vi "Measurement UI.vi"() -> ()   [LabVIEW 2024, in "Tone Generation UI.lvlib"]
uses:
  Tone Generation UI.lvlib
  <vilib>/Utility/error.llb/Trim Whitespace One-Sided.vi
panel:
  in  "sample rate":dbl=51200.0 min=100.0 max=1000000.0 step=100.0 format="%#_g Hz"
  in  "physical channels":string[](array[string])
  in  "phases":dbl[](array[numeric])
  in  "amplitudes":dbl[](array[numeric])
  in  "frequencies":dbl[](array[numeric])
  in  "terminal cfgs":i32[](array[numeric])
  in  "ranges":dbl[](array[numeric])
  in  "output configurations":T1(array[cluster])=[{"channel"="Dev1/ao0", "range"=3.16, "terminal configuration"=-1, "frequency"=997.0, "amplitude"=1.0, "phase"=0.0}, {"channel"="Dev1/ao1", "range"=3.16, "terminal configuration"=-1, "frequency"=997.0, "amplitude"=1.0, "phase"=90.0}] {"phase" min=-360.0 max=360.0 step=10.0 format="%#_g deg"; "amplitude" min=0.0 max=10.0 format="%_4g V"; "frequency" min=0.001 step=10.0 format="%#_4g Hz"; "terminal configuration" items=["Default"=-1, "RSE"=10083, "Differential"=10106, "Pseudodifferential"=12529]; "range" min=0.1 max=10.0 step=1.0 format="± %#_4g V"}
  out "error code out":i32
  out "error description out":string="Empty"
  out "error out":bool
  out "Task":u16(ring)
  out "generator status":string="Idle"
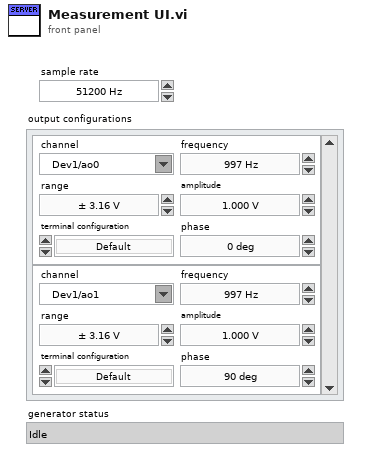
[diagram p1: front panel]
types:
  T1 = cluster{"channel":tag, "range":dbl, "terminal configuration":i32, "frequency":dbl, "amplitude":dbl, "phase":dbl}[]
  T2 = cluster{"channel":tag, "range":dbl, "terminal configuration":i32, "frequency":dbl, "amplitude":dbl, "phase":dbl}
  T3 = enum8{"Enabled", "Disabled", "Disabled and Grayed Out"}
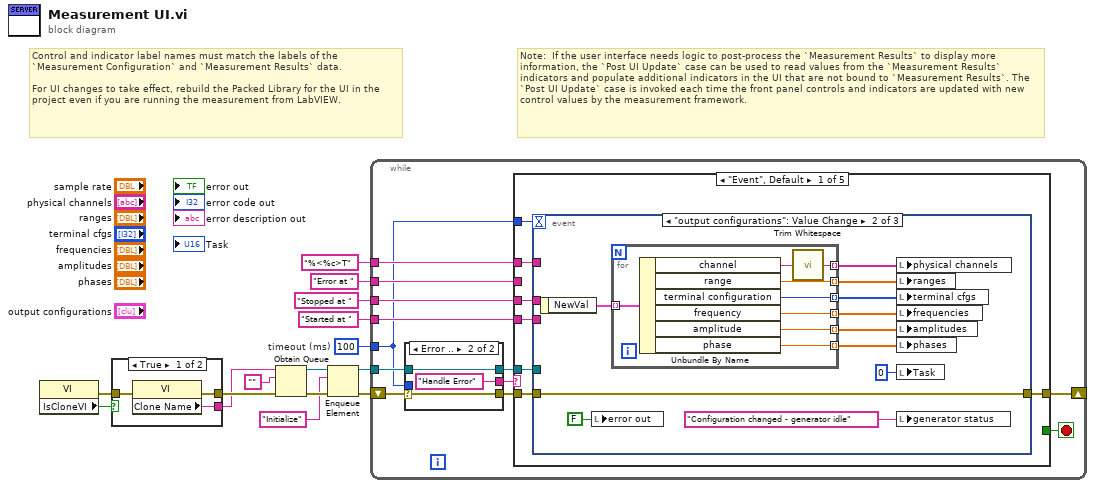
[diagram p0: block diagram]
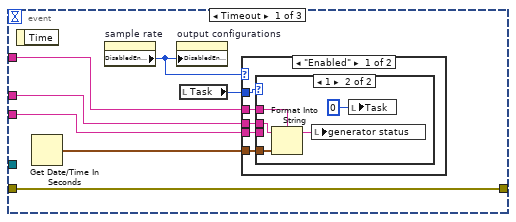
[diagram p2: hidden frame]
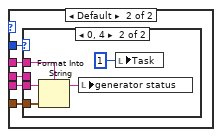
[diagram p4: hidden frame]
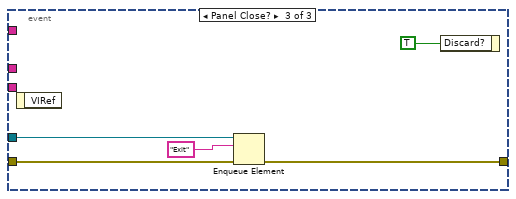
[diagram p6: hidden frame]
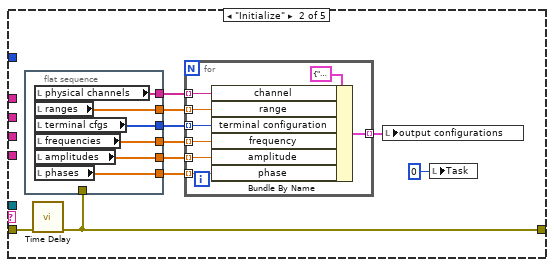
[diagram p7: hidden frame]
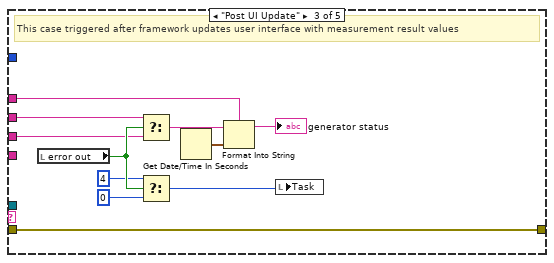
[diagram p8: hidden frame]
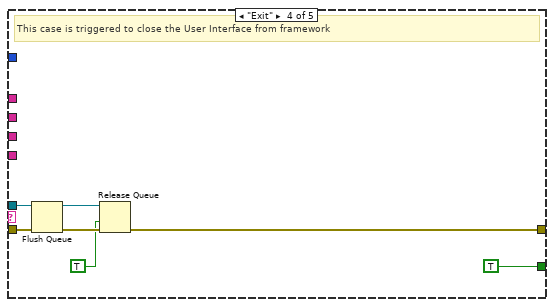
[diagram p9: hidden frame]
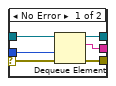
[diagram p11: hidden frame]
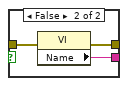
[diagram p12: hidden frame]
diagram:
  w1 = 100  # timeout (ms)
  # "Control and indicator label names must match the labels of the `Measurement Configuration` and `Measurement Results` data. \n\nFor UI changes to take effect, rebuild the Packed Library for the UI in the project even if you are running the measurement from LabVIEW."
  # "Note:  If the user interface needs logic to post-process the `Measurement Results` to display more information, the `Post UI Update` case can be used to read values from the `Measurement Results` indicators and populate additional indicators in the UI that are not bound to `Measurement Results`. The `Post UI Update` case is invoked each time the front panel controls and indicators are updated with new control values by the measurement framework."
  n1 = property class="VI"() -> (error out=w6:errorcluster, "IsCloneVI"=w7:bool)  [unwired: 2 in, 1 out]
  n2 = case shown="True" w7 {
    tunnel: [w18 w21] -> w15
    tunnel: [w17 w20] -> w14
    tunnel: w6 -> [w16 w19]
    frame True {
      n3 = property class="VI"(error in=w16) -> (error out=w18:errorcluster, "Clone Name"=w17:string)  [unwired: 1 in, 1 out]
    }
    frame False {
      n4 = property class="VI"(error in=w19) -> (error out=w21:errorcluster, "Name"=w20:string)  [unwired: 1 in, 1 out]
    }
  }
  n5 = Obtain Queue(name (unnamed)=w14, element data type="", error in (no error)=w15) -> (queue out=w11:refnum<queue>, error out=w13:errorcluster)  [unwired: 2 in, 1 out]
  n6 = Enqueue Element(queue=w11, element="Initialize", error in (no error)=w13) -> (queue out=w10:refnum<queue>, error out=w12:errorcluster)  [unwired: 1 in, 1 out]
  n7 = while {
    shift-right: [w28] -> _
    shift-left: w12 -> [w33]
    tunnel: w10 -> [w31]
    tunnel: "Started at " ("format string") -> [w26]
    tunnel: "Error at " ("current status") -> [w25]
    tunnel: "Stopped at " ("current status") -> [w24]
    tunnel: "%<%c>T" ("format string") -> [w23]
    tunnel: w1 -> [w22]
    stop <- w27 stop-if-true
    n8 = case shown="Error .." w33 {
      selector: w33 -> [w140 w143]
      tunnel: [w139 w143] -> w32
      tunnel: w31 -> [w138 w142]
      tunnel: [w137 w142] -> w30
      tunnel: [w136 "Handle Error"] -> w29
      tunnel: w22 -> [w135 _]
      frame No Error {
        n9 = Dequeue Element(queue=w138, timeout in ms (-1)=w135, error in (no error)=w140) -> (queue out=w137:refnum<queue>, element=w136:string, error out=w139:errorcluster)  [unwired: 1 out]
      }
      frame Error {
      }
    }
    n10 = case shown="\"Event\", Default" w29 {
      tunnel: w32 -> [w39 w100 w126 w133 w134]
      tunnel: w30 -> [w38 _ _ w131 _]
      tunnel: [w40 w92 w126 w128 w134] -> w28
      tunnel: [_ _ _ TRUE _] -> w27
      tunnel: w22 -> [w37 _ _ _ _]
      tunnel: w25 -> [_ _ w118 _ _]
      tunnel: w24 -> [w35 _ w117 _ _]
      tunnel: w26 -> [w36 _ _ _ _]
      tunnel: w23 -> [w34 _ w116 _ _]
      frame "Event", Default {
        n11 = event shown="[1] \"output configurations\": Value Change" {
          selector: _ -> [_ _ _]
          dyn-events: _ -> [_ _ _]
          timeout: w37 -> [_ _ _]
          tunnel: [w47 w78 w89] -> w40
          tunnel: w39 -> [w47 w78 w90]
          tunnel: w38 -> [_ _ w88]
          tunnel: w36 -> [w44 _ _]
          tunnel: w35 -> [w42 _ _]
          tunnel: w34 -> [w41 _ _]
          event Timeout {
            n12 = event-data() -> ()  [unwired: 1 in, 1 out]
            n13 = Get Date/Time In Seconds() -> (seconds since 1Jan1904=w43:timestamp)
            n14 = property on="sample rate" class="DigNum (strict)"() -> ("DisabledEnum"=w46:T3)  [unwired: 2 in, 2 out]
            n15 = property on="output configurations" class="Arr (strict)"("DisabledEnum"=w46) -> ()  [unwired: 2 in, 2 out]
            n16 = local read "Task"() -> (w45:u16)
            n17 = case shown="\"Enabled\"" w46 {
              tunnel: w45 -> [w52 w62]
              tunnel: w44 -> [w49 w61]
              tunnel: w41 -> [w51 w59]
              tunnel: w43 -> [w50 w60]
              tunnel: w42 -> [w48 w58]
              frame "Enabled" {
                n18 = case shown="1" w52 {
                  tunnel: w51 -> [_ w55]
                  tunnel: w50 -> [_ w54]
                  tunnel: w49 -> [_ _]
                  tunnel: w48 -> [_ w53]
                  frame Default {
                  }
                  frame 1 {
                    n19 = Format Into String(format string=w55, initial string=w53, w54) -> (resulting string=w57:string)  [unwired: 1 in, 1 out]
                    n20 = local write "generator status"(w57) -> ()
                    n21 = local write "Task"(u16 0 ("Task")) -> ()
                  }
                }
              }
              frame Default {
                n22 = case shown="0, 4" w62 {
                  tunnel: w61 -> [_ w65]
                  tunnel: w60 -> [_ w64]
                  tunnel: w59 -> [_ w63]
                  tunnel: w58 -> [_ _]
                  frame Default {
                  }
                  frame 0, 4 {
                    n23 = Format Into String(format string=w63, initial string=w65, w64) -> (resulting string=w67:string)  [unwired: 1 in, 1 out]
                    n24 = local write "generator status"(w67) -> ()
                    n25 = local write "Task"(u16 1 ("Task")) -> ()
                  }
                }
              }
            }
          }
          event "output configurations": Value Change {
            n26 = event-data() -> ("NewVal"=w71:T1)  [unwired: 1 in]
            n27 = local write "error out"(FALSE ("error out")) -> ()
            n28 = for {
              tunnel: w71 -> [w86] mode=indexing
              tunnel: [w79] -> w77 mode=indexing
              tunnel: [w85] -> w76 mode=indexing
              tunnel: [w84] -> w75 mode=indexing
              tunnel: [w83] -> w74 mode=indexing
              tunnel: [w82] -> w73 mode=indexing
              tunnel: [w81] -> w72 mode=indexing
              n29 = Unbundle By Name(w86) -> ("channel"=w80:tag, "range"=w85:dbl, "terminal configuration"=w84:i32, "frequency"=w83:dbl, "amplitude"=w82:dbl, "phase"=w81:dbl)
              n30 = call <vilib>:"Trim Whitespace.vi"("string"=w80) -> ("trimmed string"=w79:string)  [unwired: 1 in]
            }
            n31 = local write "physical channels"(w77) -> ()
            n32 = local write "ranges"(w76) -> ()
            n33 = local write "terminal cfgs"(w75) -> ()
            n34 = local write "frequencies"(w74) -> ()
            n35 = local write "amplitudes"(w73) -> ()
            n36 = local write "phases"(w72) -> ()
            n37 = local write "Task"(u16 0 ("Task")) -> ()
            n38 = local write "generator status"("Configuration changed - generator idle" ("current status")) -> ()
          }
          event Panel Close? {
            n39 = event-data() -> ()  [unwired: 1 in, 1 out]
            n40 = Enqueue Element(queue=w88, element="Exit", error in (no error)=w90) -> (error out=w89:errorcluster)  [unwired: 1 in, 2 out]
            n41 = event-data("Discard?"=TRUE) -> ()  [unwired: 1 in, 1 out]
          }
        }
      }
      frame "Initialize" {
        n42 = flat-sequence {
          tunnel: [w107] -> w99
          tunnel: [w106] -> w98
          tunnel: [w105] -> w97
          tunnel: [w104] -> w96
          tunnel: [w103] -> w95
          tunnel: [w102] -> w94
          tunnel: w92 -> [_]
          frame #0 {
            n43 = local read "physical channels"() -> (w107:string[])
            n44 = local read "ranges"() -> (w106:dbl[])
            n45 = local read "terminal cfgs"() -> (w105:i32[])
            n46 = local read "frequencies"() -> (w104:dbl[])
            n47 = local read "amplitudes"() -> (w103:dbl[])
            n48 = local read "phases"() -> (w102:dbl[])
          }
        }
        n49 = call "Time Delay"("error in (no error)"=w100) -> ("error out"=w92:errorcluster)  [unwired: 10 in]
        n50 = for {
          tunnel: w99 -> [w115] mode=indexing
          tunnel: w98 -> [w114] mode=indexing
          tunnel: w97 -> [w113] mode=indexing
          tunnel: w96 -> [w112] mode=indexing
          tunnel: w95 -> [w111] mode=indexing
          tunnel: w94 -> [w110] mode=indexing
          tunnel: [w108] -> w93 mode=indexing
          n51 = Bundle By Name(cluster=T2 {"channel"="Dev1/ao0", "range"=3.16, "terminal configuration"=-1, "frequency"=997.0, "amplitude"=1.0, "phase"=0.0} ("output configuration"), "channel"=w115, "range"=w114, "terminal configuration"=w113, "frequency"=w112, "amplitude"=w111, "phase"=w110) -> (w108:T2)
        }
        n52 = local write "output configurations"(w93) -> ()
        n53 = local write "Task"(u16 0 ("Task")) -> ()
      }
      frame "Post UI Update" {
        # "This case triggered after framework updates user interface with measurement result values"
        n54 = local read "error out"() -> (w122:bool)
        n55 = Select(t=w118, s=w122, f=w117) -> (s? t:f=w125:string)
        n56 = Select(t=u16 4 ("Task"), s=w122, f=u16 0 ("Task")) -> (s? t:f=w119:u16)
        n57 = Get Date/Time In Seconds() -> (seconds since 1Jan1904=w123:timestamp)
        n58 = Format Into String(format string=w116, initial string=w125, w123) -> (resulting string=→"generator status":string)  [unwired: 1 in, 1 out]
        n59 = local write "Task"(w119) -> ()
      }
      frame "Exit" {
        # "This case is triggered to close the User Interface from framework"
        n60 = Flush Queue(queue=w131, error in (no error)=w133) -> (queue out=w130:refnum<queue>, error out=w129:errorcluster)  [unwired: 1 out]
        n61 = Release Queue(queue=w130, force destroy? (F)=TRUE, error in (no error)=w129) -> (error out=w128:errorcluster)  [unwired: 2 out]
      }
      frame "Handle Error" {
      }
    }
  }
